vi "custom init.vi"(11 "state":T1) -> (0 "abort code":i32, 3 "state out":T1)   [LabVIEW 2015, in "Scriptable Model Interface Engine.lvlib"]
uses:
  Scriptable Model Interface Engine.lvlib
  runtime state.ctl
  Shared/model parameters.ctl
  Shared/Scriptable Model Interface Shared.lvlib
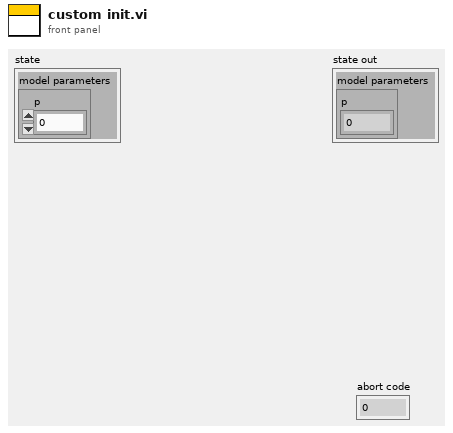
[diagram p1: front panel]
types:
  T1 = typedef "Scriptable Model Interface Engine.lvlib/runtime state.ctl" = cluster{"model parameters":T2}
  T2 = typedef "Scriptable Model Interface Shared.lvlib/model parameters.ctl" = cluster{"p":dbl}
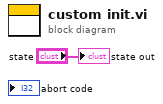
[diagram p0: block diagram]
diagram:
  "state out" <- "state"
